vi "Initialize Hdwr Interfaces.vi"(4 "error in (no error)":errorcluster, 7 "Instance Name":T1) -> (0 "error out":errorcluster)   [LabVIEW 2015, in "Startup Processes.lvlib"]
uses:
  Startup Processes.lvlib
  _typedefs/Subpanel Names.ctl
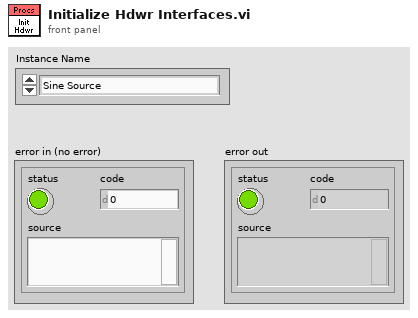
[diagram p1: front panel]
types:
  T1 = typedef "Startup Processes.lvlib/Subpanel Names.ctl" = enum16{"Sine Source", "Ramp Source", "Hen House TC", "Dog House TC", "Out House TC"}
  T2 = enum16{"Write Fan State", "Write Cooler State", "Read"}
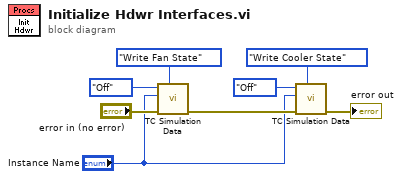
[diagram p0: block diagram]
diagram:
  n1 = call "TC Simulation Data.vi"("Function"=T2."Write Fan State", "error in (no error)"="error in (no error)", "Machine Name"="Instance Name", "State In"=enum16{"Off", "On"}."Off") -> ("error out"=w8:errorcluster)  [unwired: 2 in, 2 out]
  n2 = call "TC Simulation Data.vi"("Function"=T2."Write Cooler State", "error in (no error)"=w8, "Machine Name"="Instance Name", "State In"=enum16{"Off", "On"}."Off") -> ("error out"=→"error out":errorcluster)  [unwired: 2 in, 2 out]
